vi "Pick.vi"(4 "Side":T1=enum."right", 9 "Part Name":string="Large Gear", 11 "Location":T2={"x"=50.0, "y"=900.0, "a"=900.0, "Name"="Large Gear"}) -> (0 "error out":errorcluster)   [LabVIEW 2013]
uses:
  Move/Move Reference.vi
  Move/Move Matrix.vi
  ROS/Code/SubVIs/BaxterSide.ctl
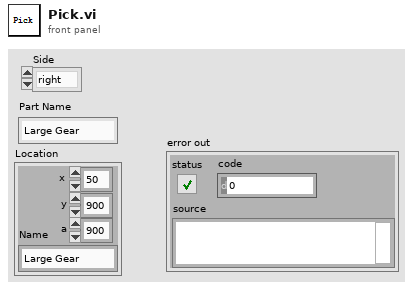
[diagram p1: front panel]
types:
  T1 = typedef "BaxterSide.ctl" = enum16{"left", "right"}
  T2 = cluster{"x":dbl, "y":dbl, "a":dbl, "Name":string}
  T3 = cluster{"X":dbl, "Y":dbl, "Z":dbl, "O":dbl, "A":dbl, "T":dbl}
  T4 = typedef "NI_Matrix.lvlib/RealMatrix.ctl" = dbl[][]
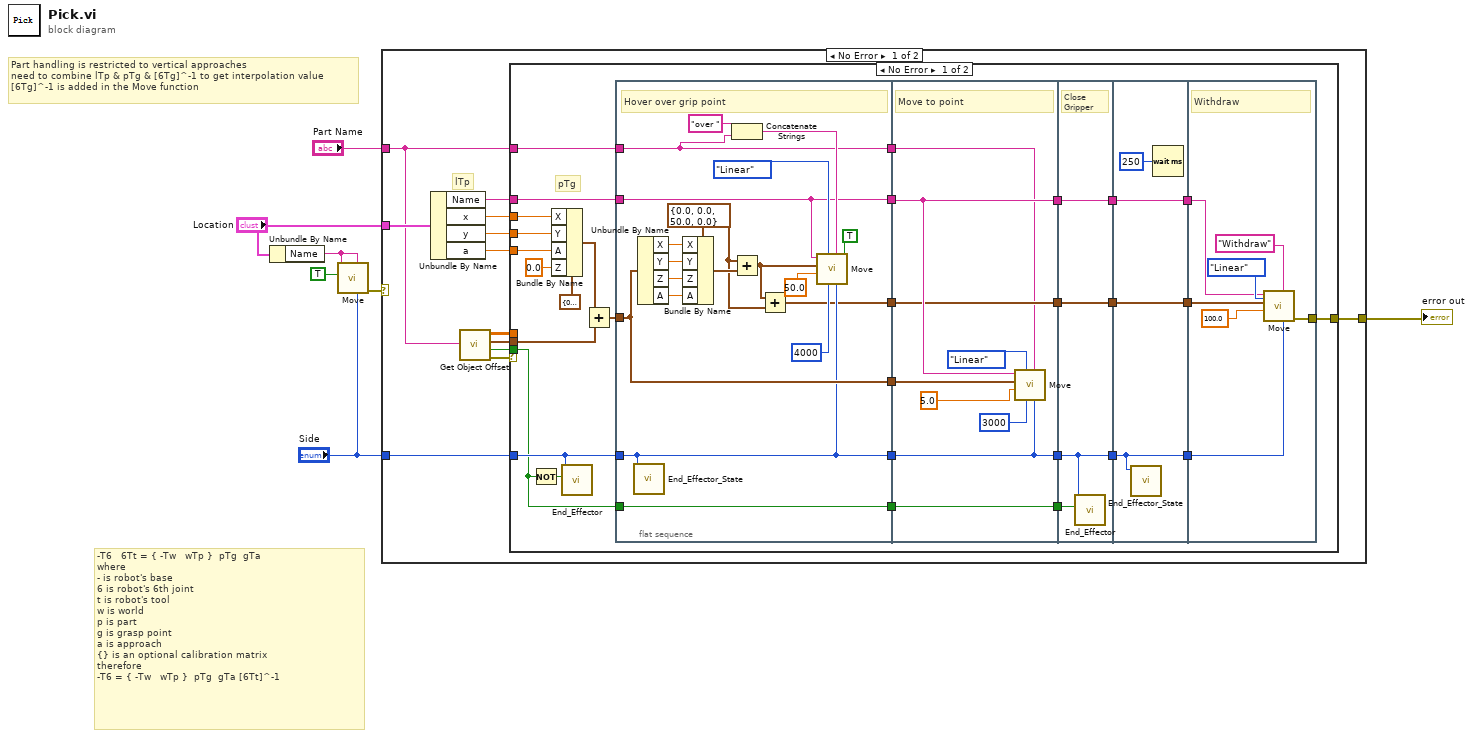
[diagram p0: block diagram]
diagram:
  # "Part handling is restricted to vertical approaches\nneed to combine lTp & pTg & [6Tg]^-1 to get interpolation value\n[6Tg]^-1 is added in the Move function"
  # "-T6   6Tt = { -Tw   wTp }  pTg  gTa\nwhere \n- is robot's base\n6 is robot's 6th joint\nt is robot's tool\nw is world\np is part\ng is grasp point\na is approach\n{} is an optional calibration matrix\ntherefore\n-T6 = { -Tw   wTp }  pTg  gTa [6Tt]^-1"
  n1 = Unbundle By Name("Location") -> ("Name"=w3:string)
  n2 = call-poly "Move.vi"("Side"="Side", "Label"=w3, "To Reference"=TRUE, "Object"=w3) -> ("error out"=w5:errorcluster)  [unwired: 7 in]
  n3 = case shown="No Error" w5 {
    selector: w5 -> [_ w94]
    tunnel: [w19 w94] -> w7
    tunnel: "Location" -> [w13 _]
    tunnel: "Side" -> [w15 _]
    tunnel: "Part Name" -> [w8 _]
    frame No Error {
      # "lTp"
      n4 = Unbundle By Name(w13) -> ("Name"=w12:string, "x"=w11:dbl, "y"=w10:dbl, "a"=w9:dbl)
      n5 = call "Get Object Offset.vi"("Label"=w8) -> ("error out"=w17:errorcluster, "GraspClose"=w16:bool, "XYZOAT"=w14:T3, "T"=w18:T4)  [unwired: 7 in]
      n6 = case shown="No Error" w17 {
        selector: w17 -> [_ w93]
        tunnel: [w49 w93] -> w19
        tunnel: w18 -> [_ _]
        tunnel: w16 -> [w20 _]
        tunnel: w15 -> [w25 _]
        tunnel: w14 -> [w47 _]
        tunnel: w12 -> [w46 _]
        tunnel: w11 -> [w45 _]
        tunnel: w10 -> [w44 _]
        tunnel: w9 -> [w43 _]
        tunnel: w8 -> [w24 _]
        frame No Error {
          # "pTg"
          n7 = Not(x=w20) -> (.not. x?=w21:bool)
          n8 = Bundle By Name(cluster=T3 {"X"=0.0, "Y"=0.0, "Z"=0.0, "O"=0.0, "A"=0.0, "T"=0.0} ("XYZOAT"), "X"=w45, "Y"=w44, "A"=w43, "Z"=0.0) -> (w48:T3)
          n9 = call "End_Effector.vi"("Close"=w21, "Side"=w25) -> ()  [unwired: 6 in, 1 out]
          n10 = Add(x=w48, y=w47) -> (x+y=w41:T3)
          n11 = flat-sequence {
            tunnel: [w55] -> w40
            tunnel: [w57] -> w39
            tunnel: [w64] -> w38
            tunnel: [w58] -> w37
            tunnel: [w52] -> w36
            tunnel: w25 -> [w55]
            tunnel: w20 -> [w57]
            tunnel: w41 -> [w64]
            tunnel: w46 -> [w58]
            tunnel: w24 -> [w54]
            tunnel: [w54] -> w23
            tunnel: w40 -> [w71]
            tunnel: [w71] -> w35
            tunnel: w39 -> [w73]
            tunnel: [w73] -> w34
            tunnel: w38 -> [w75]
            tunnel: w37 -> [w74]
            tunnel: [w74] -> w33
            tunnel: w36 -> [w72]
            tunnel: [w72] -> w32
            tunnel: w23 -> [w69]
            tunnel: w35 -> [w79]
            tunnel: [w79] -> w31
            tunnel: w34 -> [w78]
            tunnel: w33 -> [w81]
            tunnel: [w81] -> w29
            tunnel: w32 -> [w80]
            tunnel: [w80] -> w27
            tunnel: w31 -> [w82]
            tunnel: [w82] -> w30
            tunnel: w29 -> [w85]
            tunnel: [w85] -> w28
            tunnel: w27 -> [w84]
            tunnel: [w84] -> w26
            tunnel: w30 -> [w86]
            tunnel: [w92] -> w49
            tunnel: w28 -> [w87]
            tunnel: w26 -> [w88]
            frame #0 {
              w50 = cluster{"X":dbl, "Y":dbl, "Z":dbl, "A":dbl} {"X"=0.0, "Y"=0.0, "Z"=50.0, "A"=0.0} ("XYZA")
              # "Hover over grip point"
              n12 = call "End_Effector_State.vi"("Side"=w55) -> ()  [unwired: 4 in, 4 out]
              n13 = Unbundle By Name(w64) -> ("X"=w63:dbl, "Y"=w62:dbl, "Z"=w61:dbl, "A"=w60:dbl)
              n14 = Bundle By Name(cluster=w50, "X"=w63, "Y"=w62, "Z"=w61, "A"=w60) -> (w59:cluster{"X":dbl, "Y":dbl, "Z":dbl, "A":dbl})
              n15 = Concatenate Strings("over " ("string"), w54) -> (w65:string)
              n16 = Add(x=w50, y=w59) -> (x+y=w51:cluster{"X":dbl, "Y":dbl, "Z":dbl, "A":dbl})
              n17 = Add(x=w51, y=w50) -> (x+y=w52:cluster{"X":dbl, "Y":dbl, "Z":dbl, "A":dbl})
              n18 = call-poly "Move.vi"("Make Vertical"=TRUE, "Side"=w55, "Label"=w65, "Wait Time"=4000, 7:enum16{"Joint", "Linear"}."Linear" ("Motion"), "Speed (mm/s)"=50.0, "Offset"=w51, "Location"=w58) -> ()  [unwired: 3 in, 1 out]
            }
            frame #1 {
              # "Move to point"
              n19 = call-poly "Move.vi"("Side"=w71, "Label"=w69, "Wait Time"=3000 ("milliseconds to wait"), 7:enum16{"Joint", "Linear"}."Linear" ("Motion"), "Speed (mm/s)"=5.0, "Offset"=w75, "Location"=w74) -> ()  [unwired: 4 in, 1 out]
            }
            frame #2 {
              # "Close Gripper"
              n20 = call "End_Effector.vi"("Close"=w78, "Side"=w79) -> ()  [unwired: 6 in, 1 out]
            }
            frame #3 {
              n21 = call "End_Effector_State.vi"("Side"=w82) -> ()  [unwired: 4 in, 4 out]
              n22 = Wait (ms)(milliseconds to wait=u32 250) -> ()  [unwired: 1 out]
            }
            frame #4 {
              # "Withdraw"
              n23 = call-poly "Move.vi"("Side"=w86, "Label"="Withdraw", 7:enum16{"Joint", "Linear"}."Linear" ("Motion"), "Speed (mm/s)"=100.0, "Offset"=w88, "Location"=w87) -> ("error out"=w92:errorcluster)  [unwired: 5 in]
            }
          }
        }
        frame Error {
        }
      }
    }
    frame Error {
    }
  }
  "error out" <- w7
